vi "RestoreUISettings.vi"(8 "Error In":errorcluster, 11 "UI References":T1) -> (0 "Error Out":errorcluster)   [LabVIEW 2017, in "Client.lvlib" / "UI_API.lvlib"]
uses:
  UI_API.lvlib
  TypeDefs/UIReferences.ctl
  <vilib>/Utility/miscctls.llb/LVRowAndColumnTypeDef.ctl
  <vilib>/Utility/config.llb/Read Key (String).vi
  <vilib>/Utility/config.llb/Read Key (Boolean).vi
  <vilib>/Utility/config.llb/Read Key (I32).vi
  <vilib>/Utility/config.llb/NI_LVConfig.lvlib
  Client.lvlib
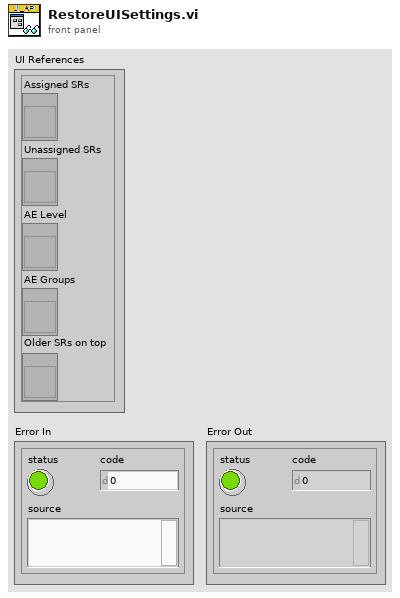
[diagram p1: front panel]
types:
  T1 = typedef "Client.lvlib/UI_API.lvlib/UIReferences.ctl" = cluster{"Assigned SRs":refnum<vi>, "Unassigned SRs":refnum<vi>, "AE Level":refnum<vi>, "AE Groups":refnum<vi>, "Older SRs on top":refnum<vi>}
  T2 = typedef "LVRowAndColumnTypeDef.ctl" = cluster{"Row":i32, "Column":i32}
  T3 = typedef "NI_LVConfig.lvlib/Config Data RefNum.ctl" = refnum<k1>
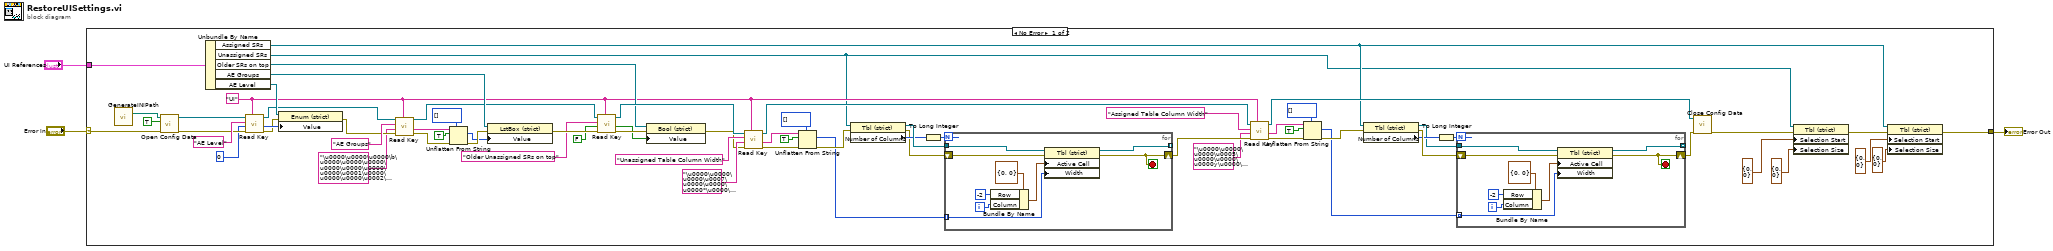
[diagram p0: block diagram]
diagram:
  n1 = case shown="No Error" "Error In" {
    selector: "Error In" -> [w71 w91]
    tunnel: "UI References" -> [w70 _]
    tunnel: [w10 w91] -> w1
    frame No Error {
      w13 = "UI" ("section")
      n2 = call "GenerateINIPath.vi"() -> ("INI Path"=w23:path)  [unwired: 11 in]
      n3 = call <vilib>:"Open Config Data.vi"("error in (no error)"=w71, "create file if necessary (T)"=TRUE ("create file if necessary? (T)"), "configuration file path"=w23) -> ("error out"=w60:errorcluster, "refnum"=w63:T3)  [unwired: 6 in, 1 out]
      n4 = Unbundle By Name(w70) -> ("Assigned SRs"=w9:refnum<vi>, "Unassigned SRs"=w4:refnum<vi>, "Older SRs on top"=w15:refnum<vi>, "AE Groups"=w68:refnum<vi>, "AE Level"=w69:refnum<vi>)
      n5 = call-poly <vilib>:"Read Key.vi"("section"=w13, "error in (no error)"=w60, "default value"=0, "key"="AE Level", "refnum"=w63) -> ("error out"=w59:errorcluster, "value"=w61:i32, "refnum out"=w55:T3)  [unwired: 3 in, 1 out]
      n6 = property class="Enum (strict)"(reference=w69, error in=w59, "Value"=w61) -> (error out=w56:errorcluster)  [unwired: 1 out]
      n7 = call-poly <vilib>:"Read Key.vi"("section"=w13, "error in (no error)"=w56, "default value"="\u0000\u0000\u0000\b\u0000\u0000\u0000\u0000\u0000\u0000\u0000\u0001\u0000\u0000\u0000\u0002\u0000\u0000\u0000\u0003\u0000\u0000\u0000\u0004\u0000\u0000\u0000\u0005\u0000\u0000\u0000\u0006\u0000\u0000\u0000\u0007", "key"="AE Groups", "refnum"=w55) -> ("error out"=w52:errorcluster, "value"=w53:string, "refnum out"=w19:T3)  [unwired: 3 in, 1 out]
      n8 = Unflatten From String(type=i32[] [] ("Value"), binary string=w53, data includes array or string size? (T)=TRUE, error in (no error)=w52) -> (value=w50:i32[], error out=w51:errorcluster)  [unwired: 1 in, 1 out]
      n9 = property class="LstBox (strict)"(reference=w68, error in=w51, "Value"=w50) -> (error out=w22:errorcluster)  [unwired: 1 out]
      n10 = call-poly <vilib>:"Read Key.vi"("section"=w13, "error in (no error)"=w22, "default value"=FALSE, "key"="Older Unassigned SRs on top", "refnum"=w19) -> ("error out"=w17:errorcluster, "value"=w14:bool, "refnum out"=w18:T3)  [unwired: 3 in, 1 out]
      n11 = property class="Bool (strict)"(reference=w15, error in=w17, "Value"=w14) -> (error out=w16:errorcluster)  [unwired: 1 out]
      n12 = call-poly <vilib>:"Read Key.vi"("section"=w13, "error in (no error)"=w16, "default value"="\u0000\u0000\u0000\u0007\u0000\u0000\u0000*\u0000\u0000\u0000F\u0000\u0000\u0000L\u0000\u0000\u0001\u0000\u0000\u0001\u0013\u0000\u0000\u0000E\u0000\u0000\u0000Z", "key"="Unassigned Table Column Width", "refnum"=w18) -> ("error out"=w45:errorcluster, "value"=w46:string, "refnum out"=w40:T3)  [unwired: 3 in, 1 out]
      n13 = Unflatten From String(type=u32[] [], binary string=w46, data includes array or string size? (T)=TRUE, error in (no error)=w45) -> (value=w43:u32[], error out=w44:errorcluster)  [unwired: 1 in, 1 out]
      n14 = property class="Tbl (strict)"(reference=w4, error in=w44) -> (reference out=w67:refnum<vi>, error out=w64:errorcluster, "Number of Columns"=w66:u32)
      n15 = To Long Integer(number=w66) -> (32bit integer=w65:i32)
      n16 = for {
        N: w65 -> [_]
        shift-right: [w84] -> w42
        shift-left: w64 -> [w85]
        tunnel: w67 -> [w90]
        tunnel: [w86] -> _ mode=indexing
        tunnel: w43 -> [w83] mode=indexing
        i -> [w82]
        stop <- w84 stop-if-true
        n17 = Bundle By Name(cluster=T2 {"Row"=0, "Column"=0} ("Active Cell:Active Cell"), "Row"=-2, "Column"=w82) -> (w87:T2)
        n18 = property class="Tbl (strict)"(reference=w90, error in=w85, "Active Cell"=w87, "Width"=w83) -> (reference out=w86:refnum<vi>, error out=w84:errorcluster)
      }
      n19 = call-poly <vilib>:"Read Key.vi"("section"=w13, "error in (no error)"=w42, "default value"="\u0000\u0000\u0000\u0005\u0000\u0000\u0000y\u0000\u0000\u0000;\u0000\u0000\u0001n\u0000\u0000\u0001\u0000\u0000\u0001\u0013", "key"="Assigned Table Column Width", "refnum"=w40) -> ("error out"=w33:errorcluster, "value"=w32:string, "refnum out"=w28:T3)  [unwired: 3 in, 1 out]
      n20 = Unflatten From String(type=u32[] [], binary string=w32, data includes array or string size? (T)=TRUE, error in (no error)=w33) -> (value=w30:u32[], error out=w31:errorcluster)  [unwired: 1 in, 1 out]
      n21 = property class="Tbl (strict)"(reference=w9, error in=w31) -> (reference out=w36:refnum<vi>, error out=w39:errorcluster, "Number of Columns"=w37:u32)
      n22 = To Long Integer(number=w37) -> (32bit integer=w38:i32)
      n23 = for {
        N: w38 -> [_]
        shift-right: [w75] -> w29
        shift-left: w39 -> [w76]
        tunnel: w36 -> [w81]
        tunnel: [w77] -> _ mode=indexing
        tunnel: w30 -> [w73] mode=indexing
        i -> [w74]
        stop <- w75 stop-if-true
        n24 = Bundle By Name(cluster=T2 {"Row"=0, "Column"=0} ("Active Cell:Active Cell"), "Row"=-2, "Column"=w74) -> (w78:T2)
        n25 = property class="Tbl (strict)"(reference=w81, error in=w76, "Active Cell"=w78, "Width"=w73) -> (reference out=w77:refnum<vi>, error out=w75:errorcluster)
      }
      n26 = call <vilib>:"Close Config Data.vi"("error in (no error)"=w29, "refnum"=w28) -> ("error out"=w12:errorcluster)  [unwired: 8 in, 1 out]
      n27 = property class="Tbl (strict)"(reference=w4, error in=w12, "Selection Start"=T2 {"Row"=0, "Column"=0}, "Selection Size"=T2 {"Row"=0, "Column"=0}) -> (error out=w11:errorcluster)  [unwired: 1 out]
      n28 = property class="Tbl (strict)"(reference=w9, error in=w11, "Selection Start"=T2 {"Row"=0, "Column"=0}, "Selection Size"=T2 {"Row"=0, "Column"=0}) -> (error out=w10:errorcluster)  [unwired: 1 out]
    }
    frame Error {
    }
  }
  "Error Out" <- w1
